vi "Calc - TBMeas.vi"(11 "01-02-9213":dbl[](array[numeric])) -> (3 "TBMeas":dbl format="%0.2f")   [LabVIEW 2018, in "Controller (Host).lvlib"]
uses:
  Controller (Host).lvlib
  <vilib>/Analysis/baseanly.llb/Mean (DBL).vi
  <vilib>/Analysis/NI_AALBase.lvlib
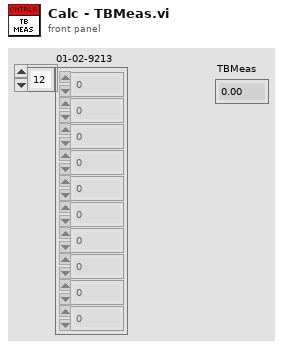
[diagram p1: front panel]
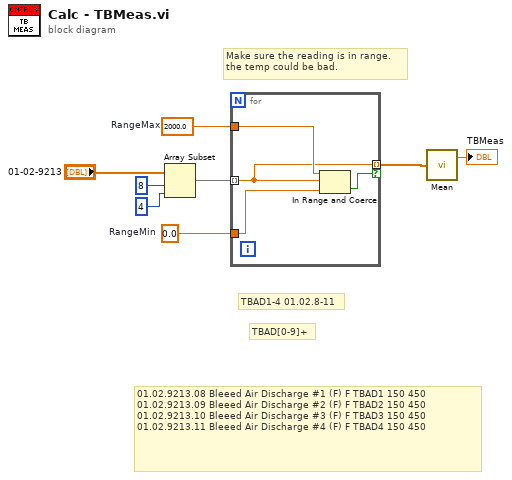
[diagram p0: block diagram]
diagram:
  w3 = 2000.0  # RangeMax
  w4 = 0.0  # RangeMin
  # "01.02.9213.08\tBleeed Air Discharge #1 (F)\tF\tTBAD1\t150\t450\n01.02.9213.09\tBleeed Air Discharge #2 (F)\tF\tTBAD2\t150\t450\n01.02.9213.10\tBleeed Air Discharge #3 (F)\tF\tTBAD3\t150\t450\n01.02.9213.11\tBleeed Air Discharge #4 (F)\tF\tTBAD4\t150\t450"
  # "TBAD[0-9]+"
  # "TBAD1-4 01.02.8-11"
  # "Make sure the reading is in range. \nthe temp could be bad."
  n1 = Array Subset(array="01-02-9213", index=8, length=4) -> (w5:dbl[])
  n2 = for {
    tunnel: w5 -> [w10] mode=indexing
    tunnel: w4 -> [w11]
    tunnel: w3 -> [w12]
    tunnel: [w10] -> w2 mode=indexing if=w9
    n3 = In Range and Coerce(upper limit=w12, x=w10, lower limit=w11) -> (In Range?=w9:bool)  [unwired: 1 out]
  }
  n4 = call-poly <vilib>:"Mean.vi"("X"=w2) -> ("mean"=→"TBMeas":dbl)  [unwired: 1 out]
